vi "HEWH End of Flow Error Check.vi"(8 "error in (no error)":errorcluster, 11 "Totalized Flow Sub-Array":dbl[](array[numeric])) -> (0 "error out":errorcluster, 3 "Sub Array End Index":i32)   [LabVIEW 2019]
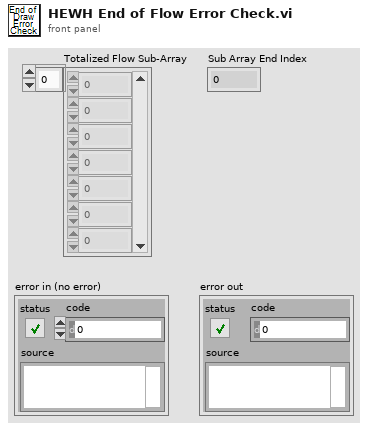
[diagram p1: front panel]
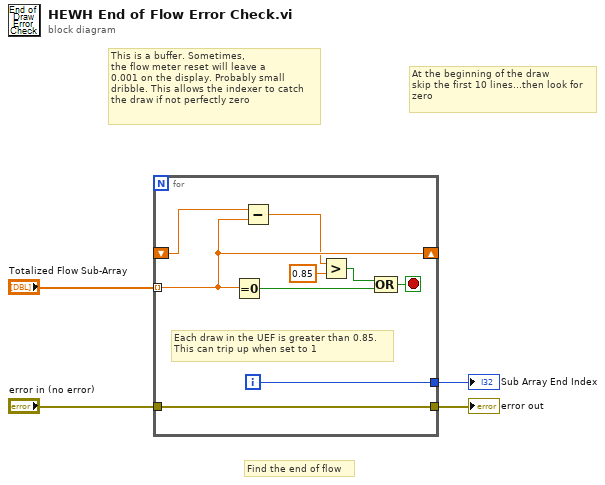
[diagram p0: block diagram]
diagram:
  # "This is a buffer. Sometimes,\nthe flow meter reset will leave a \n0.001 on the display. Probably small\ndribble. This allows the indexer to catch\nthe draw if not perfectly zero"
  # "Find the end of flow"
  # "At the beginning of the draw\nskip the first 10 lines...then look for\nzero"
  n1 = for {
    tunnel: "Totalized Flow Sub-Array" -> [w10] mode=indexing
    tunnel: [w12] -> w1
    tunnel: "error in (no error)" -> [w13]
    tunnel: [w13] -> w2
    shift-right: [w10] -> _
    shift-left: _ -> [w11]
    i -> [w12]
    stop <- w6 stop-if-true
    # "Each draw in the UEF is greater than 0.85. \nThis can trip up when set to 1"
    n2 = Equal To 0?(x=w10) -> (x = 0?=w8:bool)
    n3 = Subtract(x=w11, y=w10) -> (x-y=w5:dbl)
    n4 = Greater?(x=w5, y=0.85) -> (0:w7:bool)
    n5 = Compound Arithmetic op=OR(w7, w8) -> (w6:bool)
  }
  "error out" <- w2
  "Sub Array End Index" <- w1
